vi "LABVIEW_programming.vi"() -> ()   [LabVIEW 2022 SP3]
uses:
  <vilib>/DAQmx/write.llb/DAQmx Write (Analog DBL 1Chan 1Samp).vi
  <vilib>/DAQmx/read.llb/DAQmx Read (Analog 1D DBL NChan 1Samp).vi
  <vilib>/DAQmx/write.llb/DAQmx Write (Digital Bool 1Line 1Point).vi
  <vilib>/DAQmx/create/channels.llb/DAQmx Create Channel (AI-Voltage-Basic).vi
  <vilib>/DAQmx/create/channels.llb/DAQmx Create Channel (DO-Digital Output).vi
  <vilib>/DAQmx/create/channels.llb/DAQmx Create Channel (AO-Voltage-Basic).vi
  <vilib>/DAQmx/miscellaneous.llb/DAQmx Fill In Error Info.vi
panel:
  in  "LED Output Voltages":dbl[](array[numeric])
  out "?":i32
  out "Watering Time Complete(%)":u8(slide) scale=0.0..100.0 scale format="%.2f"
  in  "Watering Time(Min)":i32
  in  "LED controller":bool
  out "Numeric":dbl
  out "High":bool
  out "Medium":bool
  out "Low":bool
  out "Very Low":bool
  out "Pump State":bool
  out "Array":u32[](array[numeric])
  out "Light":bool
  out "Moderate":bool
  out "Dark":bool
  out "Humidity vs Time":dbl(graph)
  out "Temperature vs Time":dbl(graph)
  in  "On/Off Water Pump":bool
  out "Humidity":dbl(knob) scale=0.0..100.0
  out "Temperature":dbl(slide) scale=0.0..40.0
  in  "Stop the System":bool
  out "Humidity(RH%)":dbl format="%#_3g"
  out "Temperature(C)":dbl format="%#_3g"
  # "Grass Cutting Robot Control System"
  # "Humidity and Temperature Indicators"
  # "Pump and Water Controls"
  # "Water Tank Levels"
  # "LED Control"
  # "Light Intensity Indicators"
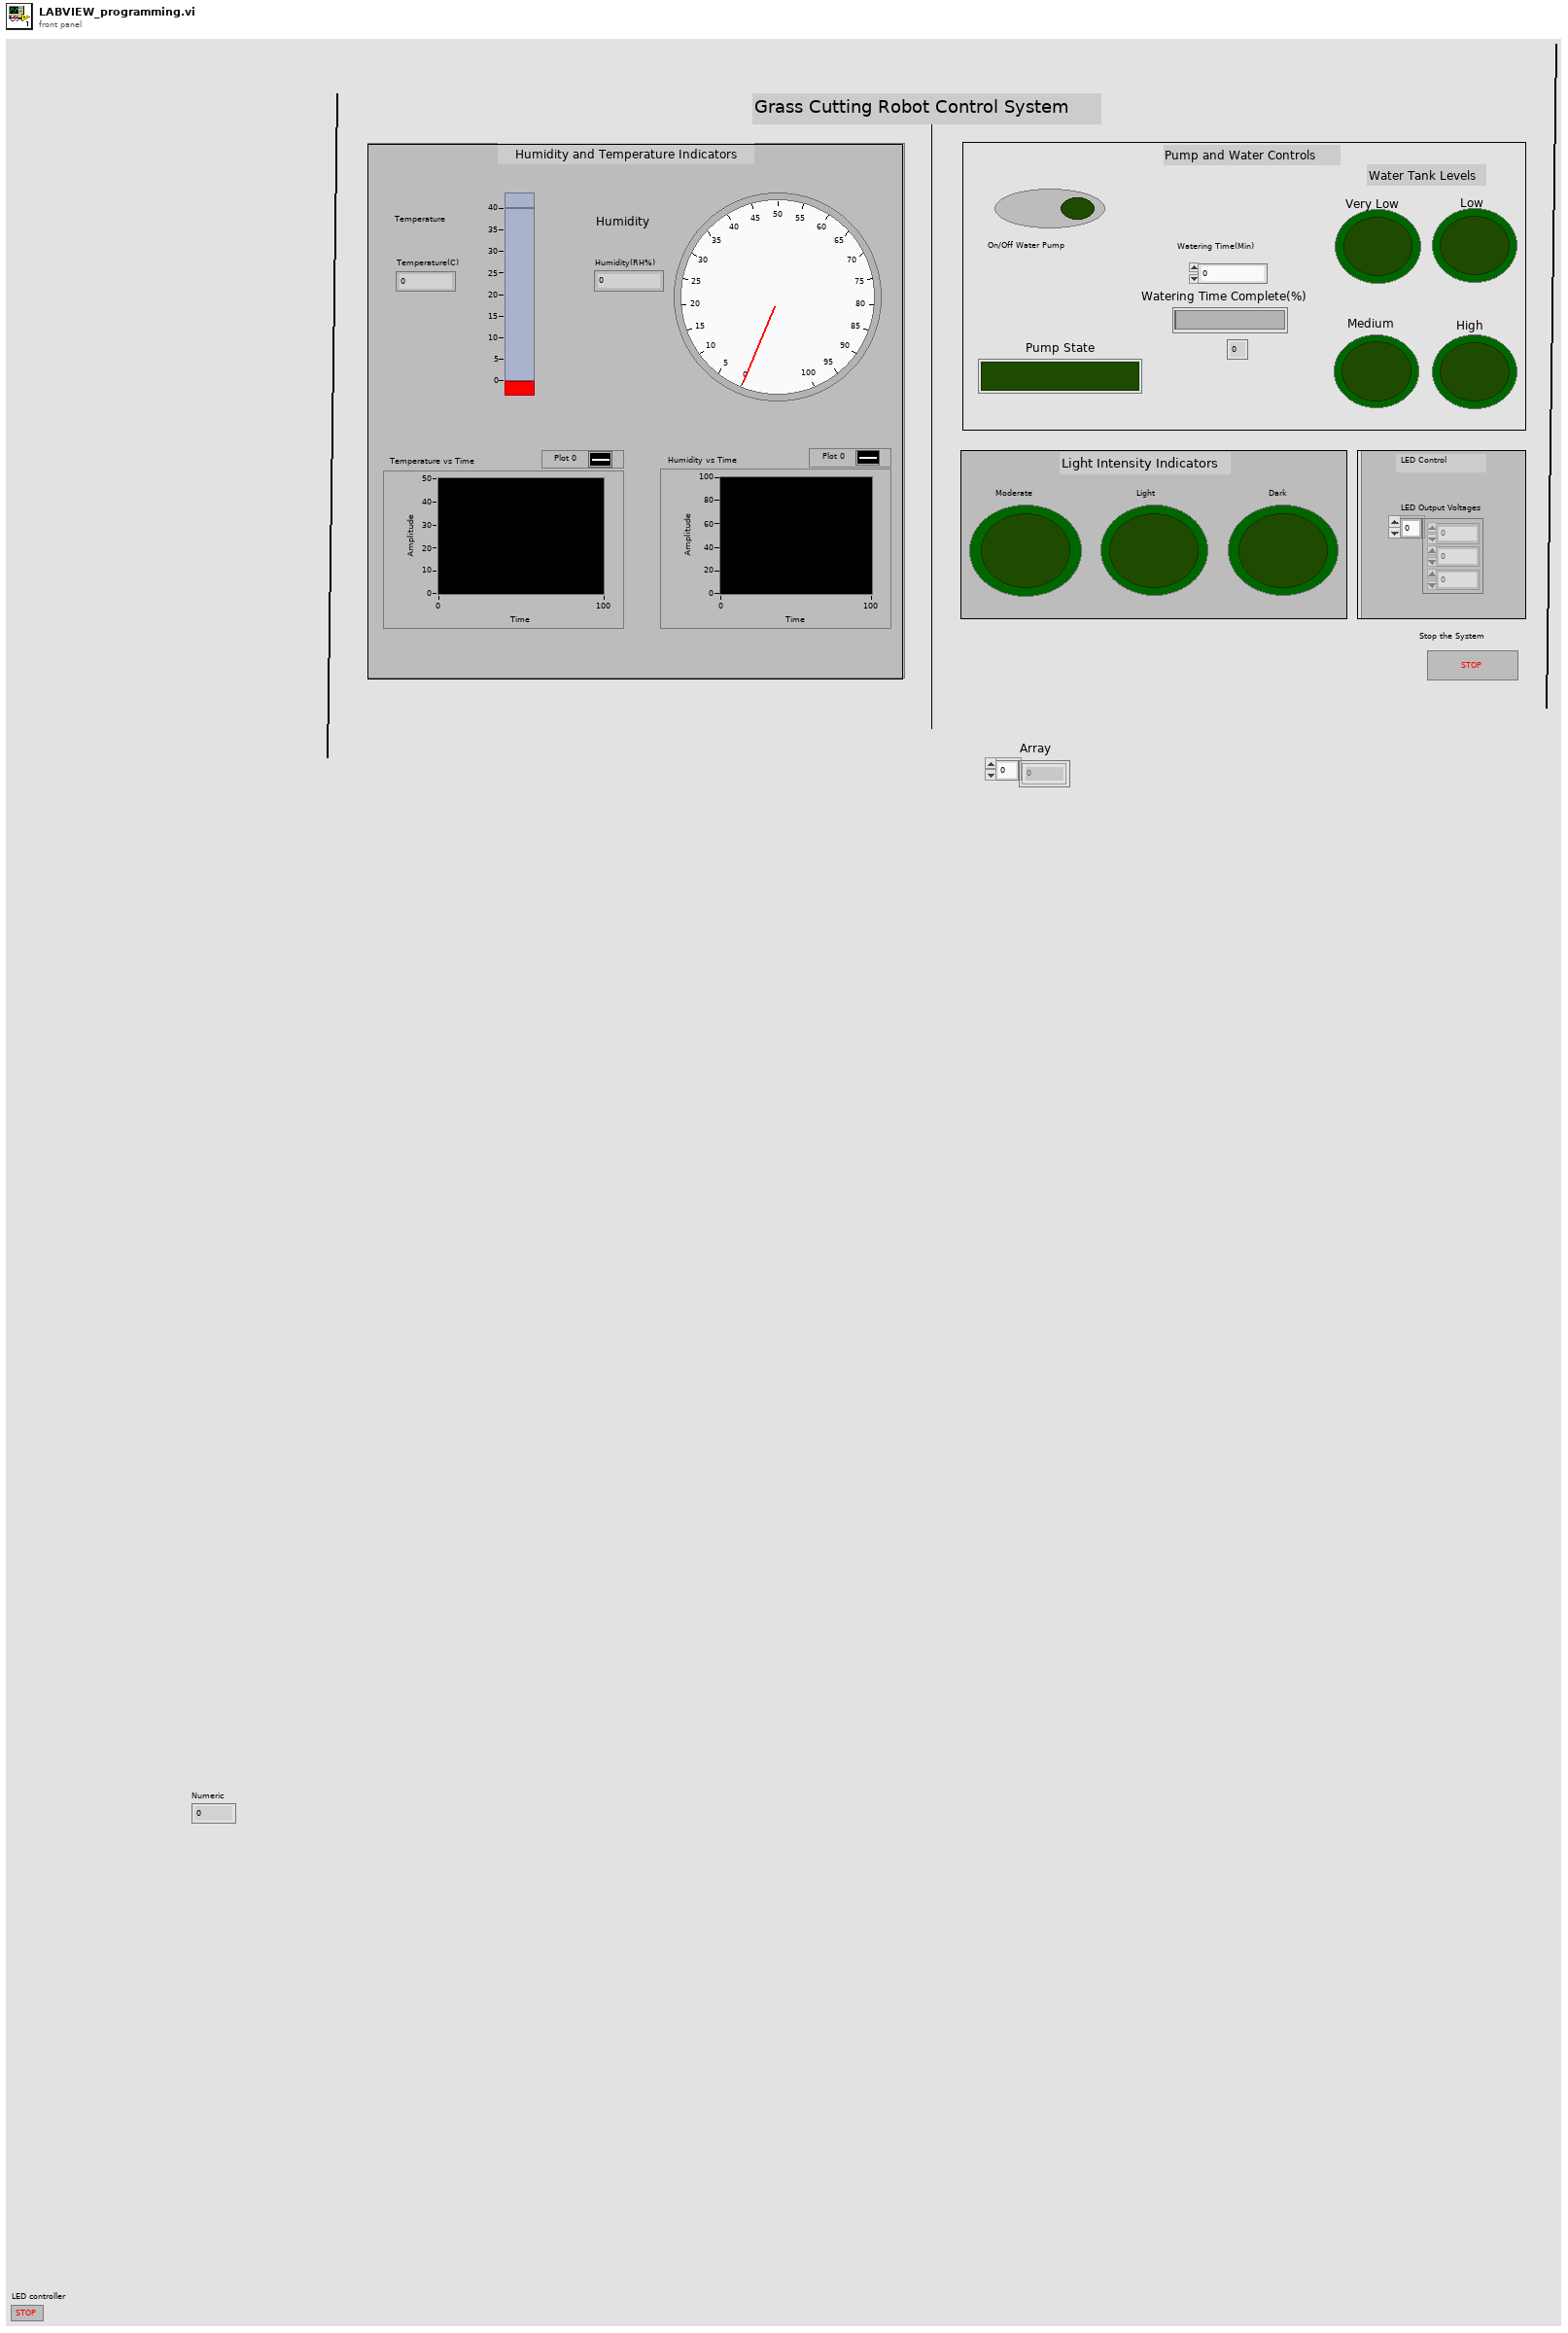
[diagram p1: front panel]
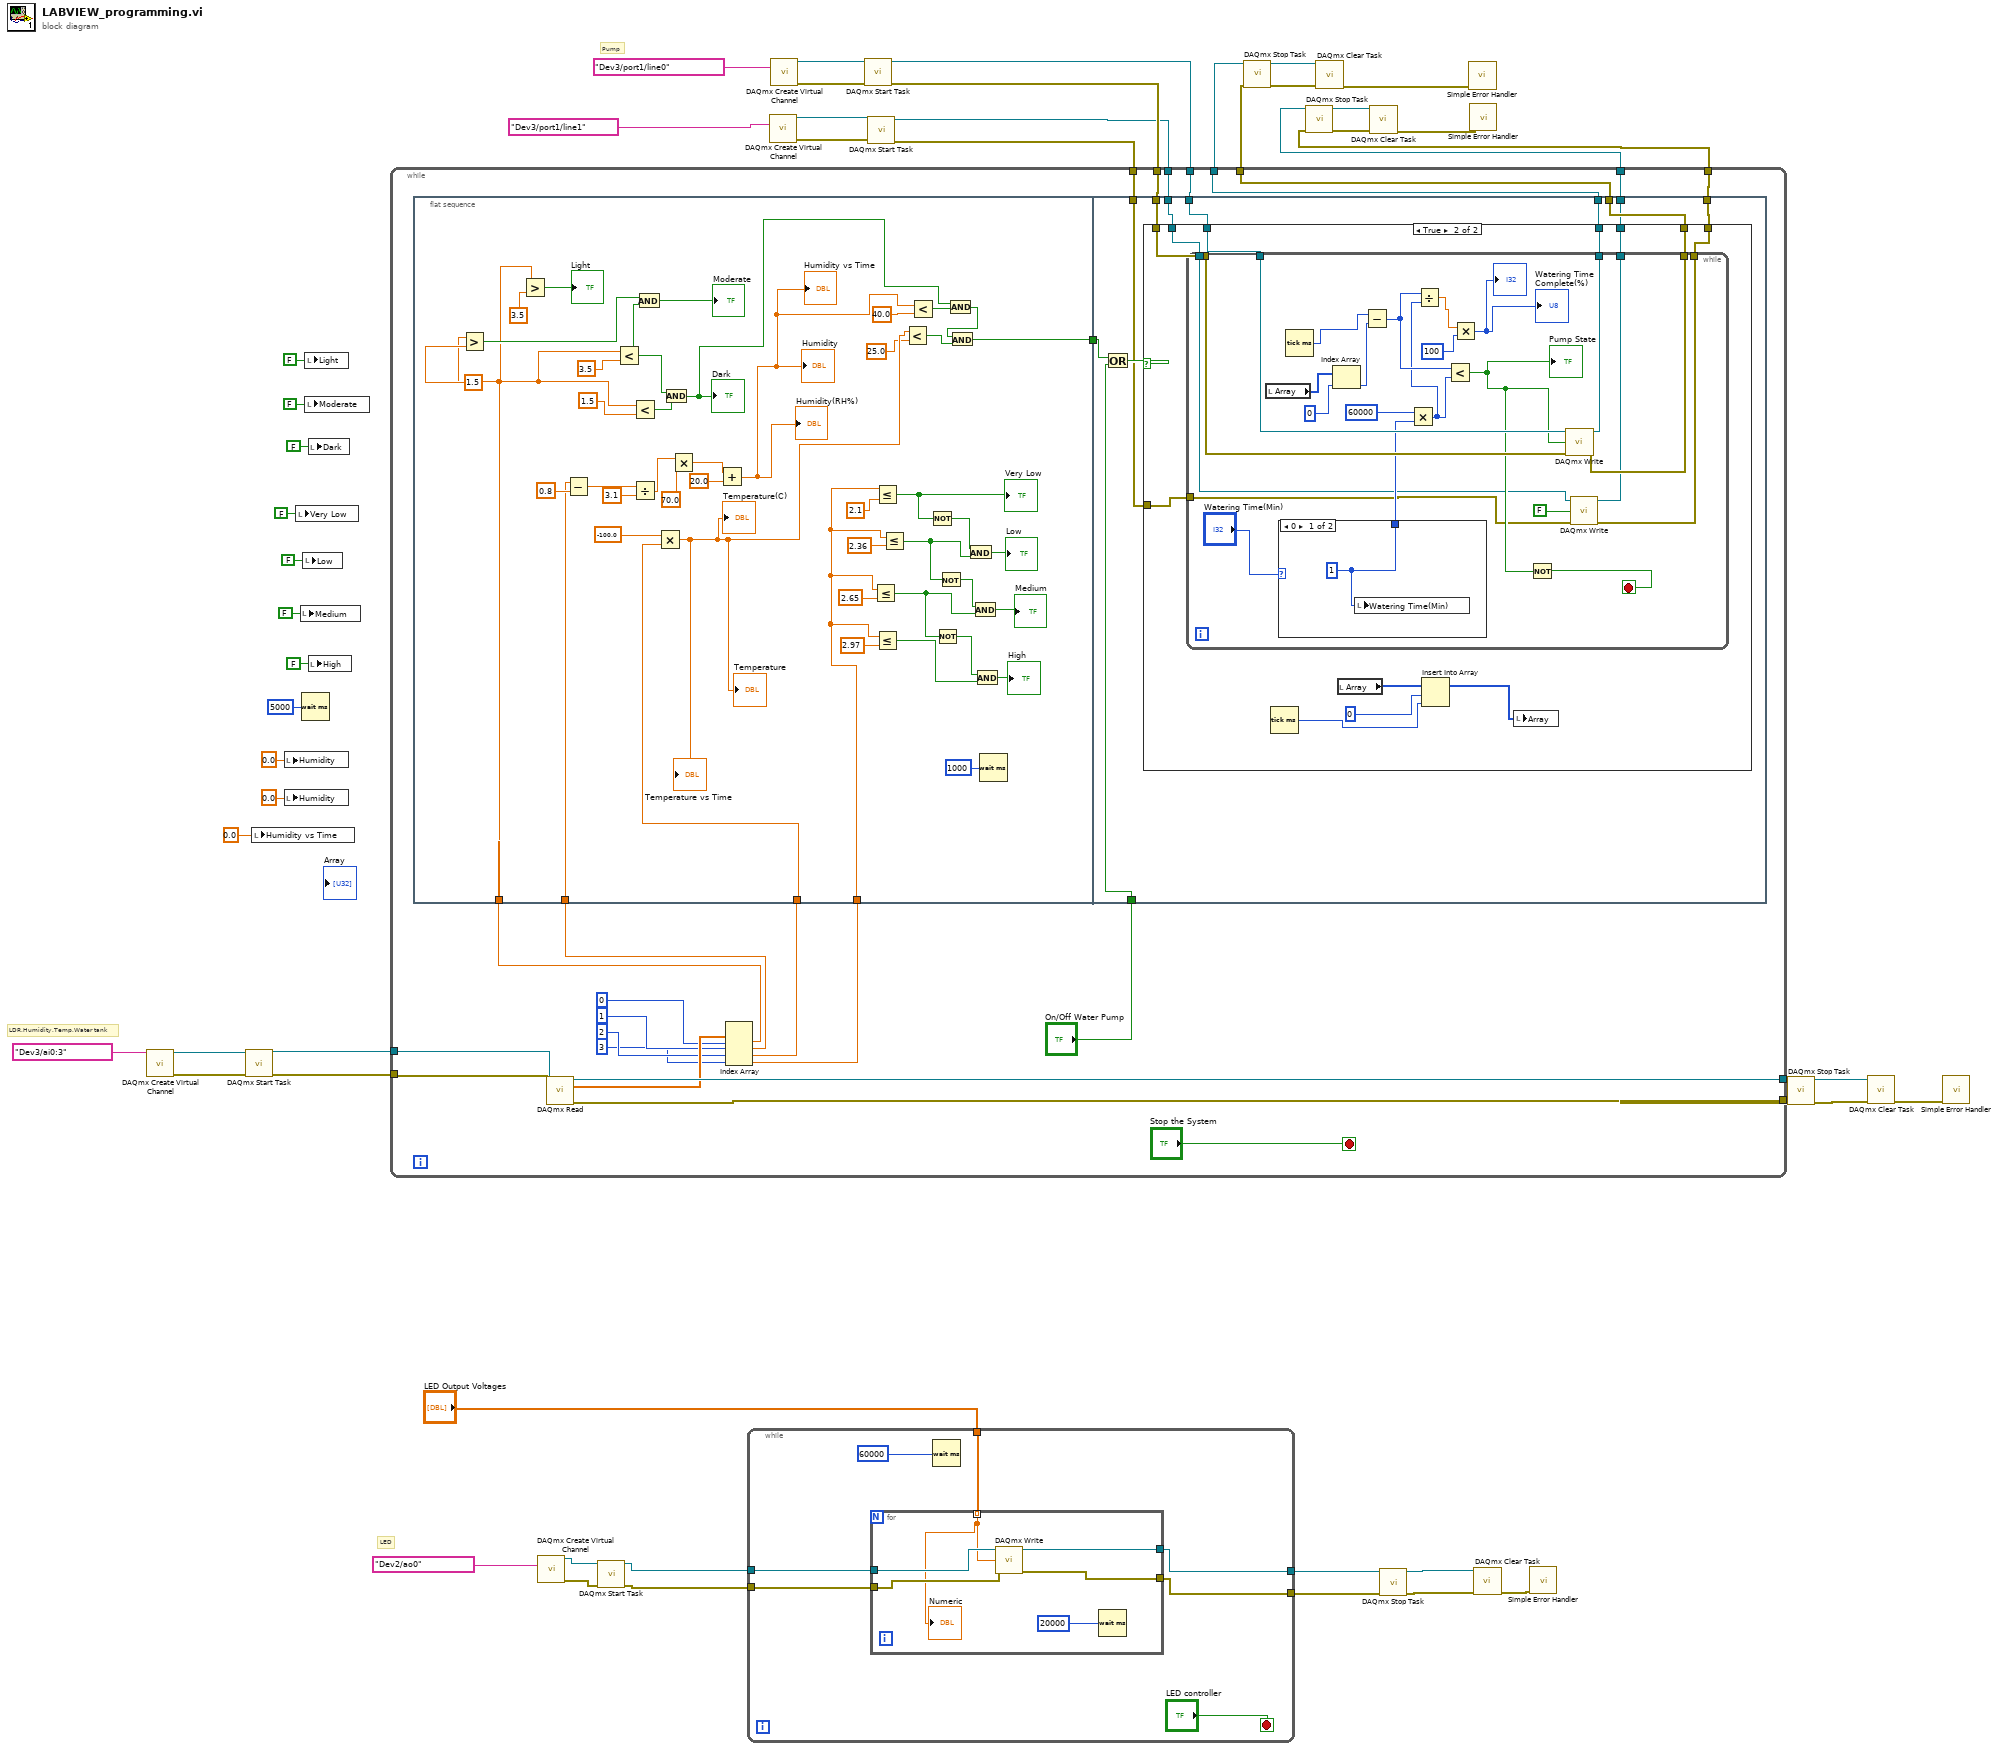
[diagram p0: block diagram]
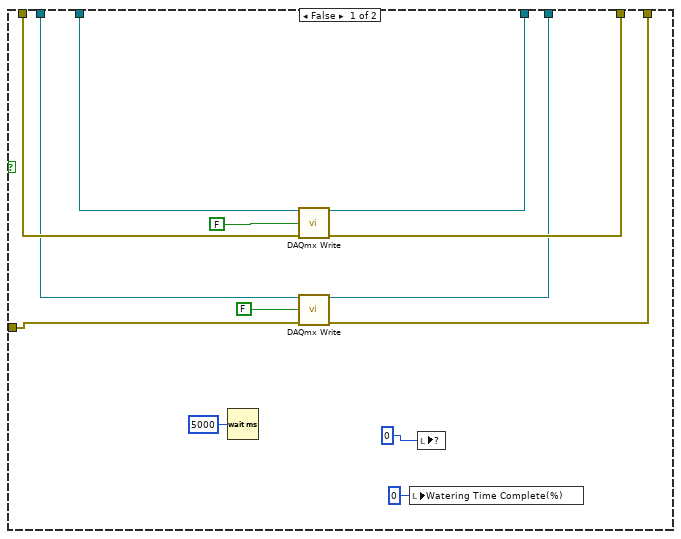
[diagram p2: hidden frame]
diagram:
  # "LED"
  # "LDR,Humidity,Temp,Water tank"
  # "Pump"
  n1 = call-poly <vilib>:"DAQmx Create Virtual Channel.vi"("physical channels"=tag "Dev3/ai0:3") -> ("task out"=w52:refnum<k21>, "error out"=w51:errorcluster)  [unwired: 13 in]
  n2 = call <vilib>:"DAQmx Start Task.vi"("task/channels in"=w52, "error in"=w51) -> ("task out"=w47:refnum<k21>, "error out"=w46:errorcluster)  [unwired: 12 in]
  n3 = local write "Humidity vs Time"(0.0 ("Humidity over Time")) -> ()
  n4 = local write "Humidity"(0.0 ("Humidity")) -> ()
  n5 = local write "Humidity"(0.0 ("Humidity")) -> ()
  n6 = local write "Very Low"(FALSE ("Very Low")) -> ()
  n7 = local write "Medium"(FALSE ("Medium")) -> ()
  n8 = Wait (ms)(milliseconds to wait=u32 5000) -> ()  [unwired: 1 out]
  n9 = local write "Low"(FALSE ("Low")) -> ()
  n10 = local write "Light"(FALSE ("Light")) -> ()
  n11 = local write "Moderate"(FALSE ("Moderate")) -> ()
  n12 = local write "Dark"(FALSE ("Dark")) -> ()
  n13 = local write "High"(FALSE ("High")) -> ()
  n14 = call-poly <vilib>:"DAQmx Create Virtual Channel.vi"("physical channels"=tag "Dev2/ao0") -> ("task out"=w32:refnum<k21>, "error out"=w31:errorcluster)  [unwired: 13 in]
  n15 = call <vilib>:"DAQmx Start Task.vi"("task/channels in"=w32, "error in"=w31) -> ("task out"=w30:refnum<k21>, "error out"=w29:errorcluster)  [unwired: 12 in]
  n16 = while {
    tunnel: w30 -> [w57]
    tunnel: w29 -> [w56]
    tunnel: [w55] -> w27
    tunnel: [w54] -> w26
    tunnel: "LED Output Voltages" -> [w53]
    stop <- "LED controller" stop-if-true
    n17 = for {
      tunnel: [w65] -> w54
      tunnel: [w63] -> w55
      tunnel: w57 -> [w62]
      tunnel: w56 -> [w61]
      tunnel: w53 -> [w60] mode=indexing
      n18 = call-poly <vilib>:"DAQmx Write.vi"("task/channels in"=w62, "data"=w60, "error in"=w61) -> ("task out"=w63:refnum<k21>, "error out"=w65:errorcluster)  [unwired: 10 in, 1 out]
      n19 = Wait (ms)(milliseconds to wait=20000) -> ()  [unwired: 1 out]
      "Numeric" <- w60
    }
    n20 = Wait (ms)(milliseconds to wait=60000) -> ()  [unwired: 1 out]
  }
  n21 = call-poly <vilib>:"DAQmx Create Virtual Channel.vi"("lines"=tag "Dev3/port1/line1" ("DAQmx Physical Channel")) -> ("task out"=w9:refnum<k21>, "error out"=w8:errorcluster)  [unwired: 13 in]
  n22 = call-poly <vilib>:"DAQmx Create Virtual Channel.vi"("lines"=tag "Dev3/port1/line0") -> ("task out"=w43:refnum<k21>, "error out"=w42:errorcluster)  [unwired: 13 in]
  n23 = call <vilib>:"DAQmx Start Task.vi"("task/channels in"=w43, "error in"=w42) -> ("task out"=w37:refnum<k21>, "error out"=w38:errorcluster)  [unwired: 12 in]
  n24 = call <vilib>:"DAQmx Start Task.vi"("task/channels in"=w9, "error in"=w8) -> ("task out"=w7:refnum<k21>, "error out"=w6:errorcluster)  [unwired: 12 in]
  n25 = while {
    tunnel: w47 -> [w89]
    tunnel: w46 -> [w88]
    tunnel: [w87] -> w45
    tunnel: [w85] -> w44
    tunnel: w38 -> [w77]
    tunnel: w37 -> [w75]
    tunnel: [w76] -> w36
    tunnel: [w74] -> w35
    tunnel: w7 -> [w69]
    tunnel: w6 -> [w68]
    tunnel: [w67] -> w5
    tunnel: [w66] -> w4
    stop <- "Stop the System" stop-if-true
    n26 = flat-sequence {
      tunnel: w82 -> [w125]
      tunnel: w81 -> [w115]
      tunnel: w78 -> [w117]
      tunnel: w71 -> [w101]
      tunnel: [w108] -> w70
      tunnel: w77 -> [w145]
      tunnel: [w144] -> w76
      tunnel: w75 -> [w143]
      tunnel: [w142] -> w74
      tunnel: "On/Off Water Pump" -> [w141]
      tunnel: w70 -> [w140]
      tunnel: w69 -> [w138]
      tunnel: w68 -> [w137]
      tunnel: [w136] -> w67
      tunnel: [w135] -> w66
      frame #0 {
        n27 = Greater?(x=w125, y=1.5) -> (0:w129:bool)
        n28 = Greater?(x=w125, y=3.5) -> (0:→"Light":bool)
        n29 = Subtract(x=w117, y=0.8) -> (x-y=w119:dbl)
        n30 = Less?(x=w125, y=3.5) -> (x < y?=w130:bool)
        n31 = Less?(x=w125, y=1.5) -> (x < y?=w132:bool)
        n32 = Divide(x=w119, y=3.1) -> (x/y=w121:dbl)
        n33 = And(x=w129, y=w130) -> (x .and. y?=→"Moderate":bool)
        n34 = Multiply(x=-100.0, y=w115) -> (x*y=w107:dbl)
        "Temperature(C)" <- w107
        "Temperature" <- w107
        "Temperature vs Time" <- w107
        n35 = And(x=w130, y=w132) -> (x .and. y?=w112:bool)
        "Dark" <- w112
        n36 = Multiply(x=w121, y=70.0) -> (x*y=w123:dbl)
        n37 = Add(x=w123, y=20.0) -> (x+y=w113:dbl)
        "Humidity(RH%)" <- w113
        "Humidity" <- w113
        "Humidity vs Time" <- w113
        n38 = Less Or Equal?(x=w101, y=2.65) -> (x <= y?=w94:bool)
        n39 = Less Or Equal?(x=w101, y=2.1) -> (x <= y?=w90:bool)
        "Very Low" <- w90
        n40 = Less Or Equal?(x=w101, y=2.97) -> (x <= y?=w93:bool)
        n41 = Less Or Equal?(x=w101, y=2.36) -> (x <= y?=w96:bool)
        n42 = Less?(x=w107, y=25.0) -> (x < y?=w109:bool)
        n43 = Less?(x=w113, y=40.0) -> (x < y?=w110:bool)
        n44 = Not(x=w90) -> (.not. x?=w91:bool)
        n45 = Not(x=w94) -> (.not. x?=w92:bool)
        n46 = Not(x=w96) -> (.not. x?=w95:bool)
        n47 = And(x=w112, y=w110) -> (x .and. y?=w111:bool)
        n48 = And(x=w111, y=w109) -> (x .and. y?=w108:bool)
        n49 = And(x=w91, y=w96) -> (x .and. y?=→"Low":bool)
        n50 = And(x=w95, y=w94) -> (x .and. y?=→"Medium":bool)
        n51 = And(x=w92, y=w93) -> (x .and. y?=→"High":bool)
        n52 = Wait (ms)(milliseconds to wait=u32 1000) -> ()  [unwired: 1 out]
      }
      frame #1 {
        n53 = Or(x=w140, y=w141) -> (x .or. y?=w139:bool)
        n54 = case shown="True" w139 {
          tunnel: w145 -> [w158 w167]
          tunnel: [w157 w169] -> w144
          tunnel: w143 -> [w156 w168]
          tunnel: [w155 w170] -> w142
          tunnel: w138 -> [w150 w162]
          tunnel: w137 -> [w149 w161]
          tunnel: [w147 w160] -> w136
          tunnel: [w146 w159] -> w135
          frame False {
            n55 = Wait (ms)(milliseconds to wait=u32 5000) -> ()  [unwired: 1 out]
            n56 = call-poly <vilib>:"DAQmx Write.vi"("task/channels in"=w156, "data"=FALSE, "error in"=w158) -> ("task out"=w155:refnum<k21>, "error out"=w157:errorcluster)  [unwired: 10 in, 1 out]
            n57 = call-poly <vilib>:"DAQmx Write.vi"("task/channels in"=w150, "data"=FALSE, "error in"=w149) -> ("task out"=w147:refnum<k21>, "error out"=w146:errorcluster)  [unwired: 10 in, 1 out]
            n58 = local write "Watering Time Complete(%)"(u8 0 ("Watering Time Complete(%)")) -> ()
            n59 = local write item#22(0) -> ()
          }
          frame True {
            n60 = while {
              tunnel: [w193] -> w170
              tunnel: [w192] -> w169
              tunnel: w168 -> [w190]
              tunnel: w167 -> [w189]
              tunnel: w162 -> [w174]
              tunnel: w161 -> [w173]
              tunnel: [w172] -> w160
              tunnel: [w171] -> w159
              stop <- w191 stop-if-true
              n61 = local read "Array"() -> (w187:u32[])
              n62 = case shown="0" "Watering Time(Min)" {
                selector: "Watering Time(Min)" -> [_ w195]
                tunnel: [w194 w195] -> w176
                frame 0 {
                  w194 = 1
                  n63 = local write "Watering Time(Min)"(w194) -> ()
                }
                frame Default {
                }
              }
              n64 = Tick Count (ms)() -> (millisecond timer value=w188:u32)
              n65 = Index Array(array=w187, index=0) -> (element=w185:u32)
              n66 = Subtract(x=w188, y=w185) -> (x-y=w182:u32)
              n67 = Multiply(x=60000, y=w176) -> (x*y=w179:i32)
              n68 = Divide(x=w182, y=w179) -> (x/y=w181:dbl)
              n69 = Less?(x=w182, y=w179) -> (x < y?=w184:bool)
              "Pump State" <- w184
              n70 = Multiply(x=w181, y=100) -> (x*y=→"Watering Time Complete(%)" →"?":i32)
              n71 = Not(x=w184) -> (.not. x?=w191:bool)
              n72 = call-poly <vilib>:"DAQmx Write.vi"("task/channels in"=w190, "data"=w184, "error in"=w189) -> ("task out"=w193:refnum<k21>, "error out"=w192:errorcluster)  [unwired: 10 in, 1 out]
              n73 = call-poly <vilib>:"DAQmx Write.vi"("task/channels in"=w174, "data"=FALSE, "error in"=w173) -> ("task out"=w172:refnum<k21>, "error out"=w171:errorcluster)  [unwired: 10 in, 1 out]
            }
            n74 = Tick Count (ms)() -> (millisecond timer value=w164:u32)
            n75 = local read "Array"() -> (w166:u32[])
            n76 = Insert Into Array(array=w166, index=0, new element=w164) -> (w163:u32[])
            n77 = local write "Array"(w163) -> ()
          }
        }
      }
    }
    n78 = call-poly <vilib>:"DAQmx Read.vi"("task/channels in"=w89, "error in"=w88) -> ("task out"=w87:refnum<k21>, "data"=w86:dbl[], "error out"=w85:errorcluster)  [unwired: 11 in]
    n79 = Index Array(array=w86, index #1=0 ("index"), index #2=1 ("index"), index #3=2, index #4=3 ("index")) -> (element #1=w82:dbl, element #2=w78:dbl, element #3=w81:dbl, element #4=w71:dbl)
  }
  n80 = call <vilib>:"DAQmx Stop Task.vi"("task/channels in"=w35, "error in"=w36) -> ("task out"=w41:refnum<k21>, "error out"=w40:errorcluster)  [unwired: 12 in]
  n81 = call <vilib>:"DAQmx Stop Task.vi"("task/channels in"=w5, "error in"=w4) -> ("task out"=w3:refnum<k21>, "error out"=w2:errorcluster)  [unwired: 12 in]
  n82 = call <vilib>:"DAQmx Clear Task.vi"("task in"=w41, "error in"=w40) -> ("error out"=w39:errorcluster)  [unwired: 13 in]
  n83 = call <vilib>:"DAQmx Clear Task.vi"("task in"=w3, "error in"=w2) -> ("error out"=w1:errorcluster)  [unwired: 13 in]
  n84 = call <vilib>:"DAQmx Stop Task.vi"("task/channels in"=w27, "error in"=w26) -> ("task out"=w25:refnum<k21>, "error out"=w24:errorcluster)  [unwired: 12 in]
  n85 = call <vilib>:"Simple Error Handler.vi"("error in (no error)"=w39) -> ()  [unwired: 4 in, 5 out]
  n86 = call <vilib>:"Simple Error Handler.vi"("error in (no error)"=w1) -> ()  [unwired: 4 in, 5 out]
  n87 = call <vilib>:"DAQmx Clear Task.vi"("task in"=w25, "error in"=w24) -> ("error out"=w28:errorcluster)  [unwired: 13 in]
  n88 = call <vilib>:"Simple Error Handler.vi"("error in (no error)"=w28) -> ()  [unwired: 4 in, 5 out]
  n89 = call <vilib>:"DAQmx Stop Task.vi"("task/channels in"=w45, "error in"=w44) -> ("task out"=w49:refnum<k21>, "error out"=w48:errorcluster)  [unwired: 12 in]
  n90 = call <vilib>:"DAQmx Clear Task.vi"("task in"=w49, "error in"=w48) -> ("error out"=w50:errorcluster)  [unwired: 13 in]
  n91 = call <vilib>:"Simple Error Handler.vi"("error in (no error)"=w50) -> ()  [unwired: 4 in, 5 out]
